vi "FT10_Semi-Auto 2 Parse Commands.vi"(11 "Semi-Auto 2 Cluster in":T1) -> (3 "appended array":T8[](array[typedef]))   [LabVIEW 2024]
uses:
  Controls/Control_Command Cluster.ctl
  Controls/Control_Semi-Auto Port.ctl
  Controls/Control_Semi-Auto Mode.ctl
  Controls/Control_Semi-Auto Cluster 2.ctl
  Controls/Control_Semi-Auto Unitherm Load.ctl
  Controls/Control_Semi-Auto Power Level.ctl
  Controls/Control_Semi-Auto Activation Duration.ctl
  Controls/Control_Semi-Auto 2 Activation Method.ctl
panel:
  out "Mode":T2
  out "Port":T6
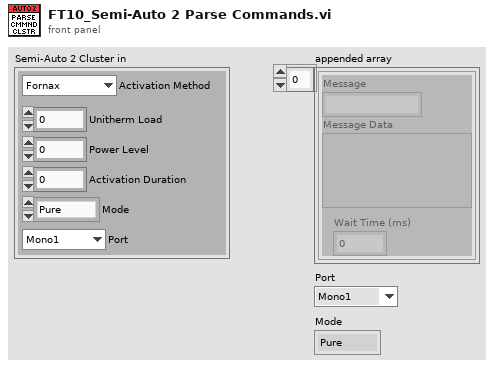
[diagram p1: front panel]
types:
  T1 = typedef "Control_Semi-Auto Cluster 2.ctl" = cluster{"Mode":T2, "Unitherm Load":T3, "Power Level":T4, "Activation Duration":T5, "Port":T6, "Activation Method":T7}
  T2 = typedef "Control_Semi-Auto Mode.ctl" = enum16{"Pure", "Blend", "Spray", "Fulgerate", "Standard", "Macro", "Precision", "Ligasure", "Error"}
  T3 = typedef "Control_Semi-Auto Unitherm Load.ctl" = i32
  T4 = typedef "Control_Semi-Auto Power Level.ctl" = dbl
  T5 = typedef "Control_Semi-Auto Activation Duration.ctl" = i32
  T6 = typedef "Control_Semi-Auto Port.ctl" = enum16{"Mono1", "Mono2", "Bipolar", "Ligasure", "Error"}
  T7 = typedef "Control_Semi-Auto 2 Activation Method.ctl" = enum16{"Fornax", "Handswitch", "Footswitch"}
  T8 = typedef "Control_Command Cluster.ctl" = cluster{"Message":string, "Message Data":variant, "Wait Time (ms)":i32}
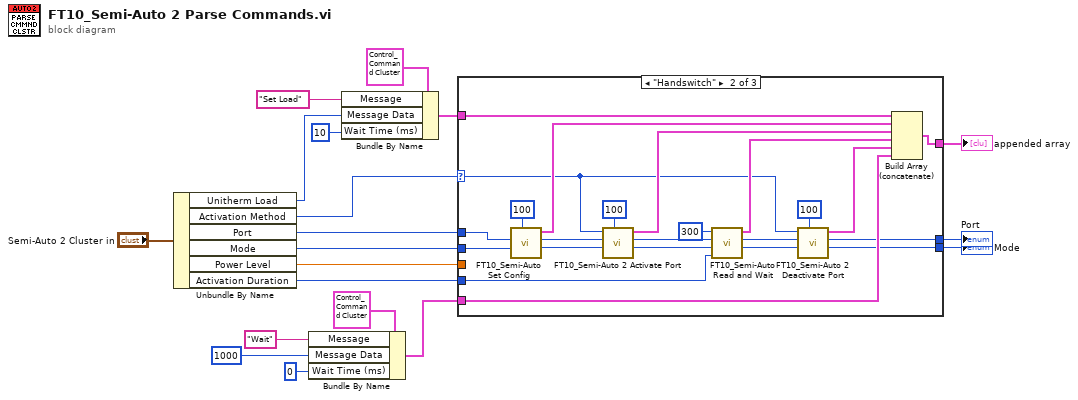
[diagram p0: block diagram]
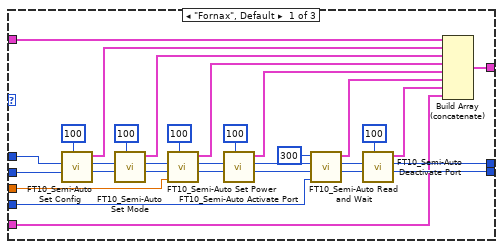
[diagram p2: hidden frame]
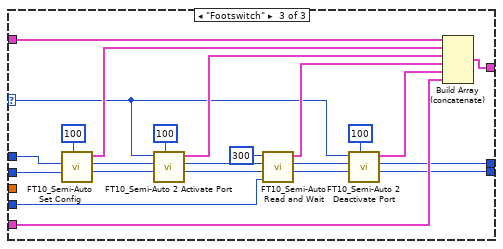
[diagram p3: hidden frame]
diagram:
  n1 = Unbundle By Name("Semi-Auto 2 Cluster in") -> ("Unitherm Load"=w15:T3, "Activation Method"=w16:T7, "Port"=w4:T6, "Mode"=w5:T2, "Power Level"=w9:T4, "Activation Duration"=w8:T5)
  n2 = Bundle By Name(cluster=T8 {"Message"="", "Message Data"=variant, "Wait Time (ms)"=0}, "Message"="Wait", "Message Data"=1000 ("Wait Time (ms)"), "Wait Time (ms)"=0) -> (w18:T8)
  n3 = Bundle By Name(cluster=T8 {"Message"="", "Message Data"=variant, "Wait Time (ms)"=0}, "Message"="Set Load", "Message Data"=w15, "Wait Time (ms)"=10) -> (w17:T8)
  n4 = case shown="\"Handswitch\"" w16 {
    selector: w16 -> [_ w52 w75]
    tunnel: w4 -> [w50 w73 w96]
    tunnel: w5 -> [w49 w72 w95]
    tunnel: [w46 w59 w82] -> w6
    tunnel: [w45 w58 w81] -> w7
    tunnel: w8 -> [w35 w69 w92]
    tunnel: w9 -> [w34 _ _]
    tunnel: w17 -> [w28 w68 w91]
    tunnel: w18 -> [w21 w62 w85]
    tunnel: [w20 w66 w89] -> w19
    frame "Fornax", Default {
      n5 = call "FT10_Semi-Auto Set Config.vi"("Wait Time (ms)"=100, "Mode in"=w49, "Port in"=w50) -> ("Mode out"=w47:T2, "Port out"=w48:T6, "output cluster"=w27:T8)  [unwired: 6 in]
      n6 = call "FT10_Semi-Auto Set Mode.vi"("Wait Time (ms)"=100, "Mode in"=w47, "Port in"=w48) -> ("Mode out"=w32:T2, "Port out"=w33:T6, "Command Cluster"=w26:T8)  [unwired: 6 in]
      n7 = call "FT10_Semi-Auto Set Power.vi"("Wait Time (ms)"=100, "Power Level"=w34, "Mode in"=w32, "Port in"=w33) -> ("Mode out"=w30:T2, "Port out"=w31:T6, "output cluster"=w25:T8)  [unwired: 5 in]
      n8 = call "FT10_Semi-Auto Activate Port.vi"("Wait Time (ms)"=100, "Mode in"=w30, "Port in"=w31) -> ("Mode out"=w41:T2, "Port out"=w40:T6, "Command Cluster"=w24:T8)  [unwired: 6 in]
      n9 = call "FT10_Semi-Auto Read and Wait.vi"("Activation Duration"=w35, "Mode in"=w41, "Port in"=w40, "Read Frequency"=300) -> ("Mode out"=w37:T2, "Port out"=w38:T6, "Command Cluster Array"=w23:T8[])  [unwired: 5 in]
      n10 = call "FT10_Semi-Auto Deactivate Port.vi"("Wait Time (ms)"=100, "Mode in"=w37, "Port in"=w38) -> ("Mode out"=w45:T2, "Port out"=w46:T6, "Command Cluster"=w22:T8)  [unwired: 6 in]
      n11 = Build Array (concatenate)(w28, w27, w26, w25, w24, w23, w22, w21) -> (w20:T8[])
    }
    frame "Handswitch" {
      n12 = call "FT10_Semi-Auto Set Config.vi"("Wait Time (ms)"=100, "Mode in"=w72, "Port in"=w73) -> ("Mode out"=w53:T2, "Port out"=w54:T6, "output cluster"=w67:T8)  [unwired: 6 in]
      n13 = call "FT10_Semi-Auto 2 Activate Port.vi"("Wait Time (ms)"=100, "Mode in"=w53, "Port in"=w54, "Activation Method in"=w52) -> ("Mode out"=w55:T2, "Port out"=w56:T6, "output cluster"=w61:T8)  [unwired: 5 in]
      n14 = call "FT10_Semi-Auto Read and Wait.vi"("Activation Duration"=w69, "Mode in"=w55, "Port in"=w56, "Read Frequency"=300) -> ("Mode out"=w57:T2, "Port out"=w60:T6, "Command Cluster Array"=w64:T8[])  [unwired: 5 in]
      n15 = call "FT10_Semi-Auto 2 Deactivate Port.vi"("Wait Time (ms)"=100, "Mode in"=w57, "Port in"=w60, "Activation Method in"=w52) -> ("Mode out"=w58:T2, "Port out"=w59:T6, "output cluster"=w63:T8)  [unwired: 5 in]
      n16 = Build Array (concatenate)(w68, w67, w61, w64, w63, w62) -> (w66:T8[])
    }
    frame "Footswitch" {
      n17 = call "FT10_Semi-Auto Set Config.vi"("Wait Time (ms)"=100, "Mode in"=w95, "Port in"=w96) -> ("Mode out"=w76:T2, "Port out"=w77:T6, "output cluster"=w90:T8)  [unwired: 6 in]
      n18 = call "FT10_Semi-Auto 2 Activate Port.vi"("Wait Time (ms)"=100, "Mode in"=w76, "Port in"=w77, "Activation Method in"=w75) -> ("Mode out"=w78:T2, "Port out"=w79:T6, "output cluster"=w84:T8)  [unwired: 5 in]
      n19 = call "FT10_Semi-Auto Read and Wait.vi"("Activation Duration"=w92, "Mode in"=w78, "Port in"=w79, "Read Frequency"=300) -> ("Mode out"=w80:T2, "Port out"=w83:T6, "Command Cluster Array"=w87:T8[])  [unwired: 5 in]
      n20 = call "FT10_Semi-Auto 2 Deactivate Port.vi"("Wait Time (ms)"=100, "Mode in"=w80, "Port in"=w83, "Activation Method in"=w75) -> ("Mode out"=w81:T2, "Port out"=w82:T6, "output cluster"=w86:T8)  [unwired: 5 in]
      n21 = Build Array (concatenate)(w91, w90, w84, w87, w86, w85) -> (w89:T8[])
    }
  }
  "appended array" <- w19
  "Port" <- w6
  "Mode" <- w7
